vi "Exam.vi"() -> ()   [LabVIEW 2018]
uses:
  <vilib>/DAQmx/write.llb/DAQmx Write (Analog Wfm 1Chan NSamp).vi
  <vilib>/DAQmx/read.llb/DAQmx Read (Analog Wfm 1Chan NSamp).vi
  <vilib>/DAQmx/create/channels.llb/DAQmx Create Channel (AI-Voltage-Basic).vi
  <vilib>/DAQmx/configure/timing.llb/DAQmx Timing (Sample Clock).vi
  <vilib>/DAQmx/miscellaneous.llb/DAQmx Fill In Error Info.vi
  <vilib>/DAQmx/create/channels.llb/DAQmx Create Channel (AO-Voltage-Basic).vi
  <vilib>/measure/NI_MABase.lvlib
panel:
  in  "정지 2":bool
  out "웨이브폼 차트 2":waveform(dbl)(graph)
  out "웨이브폼 차트":waveform(dbl)(graph)
  in  "정지":bool
  in  "정지":bool
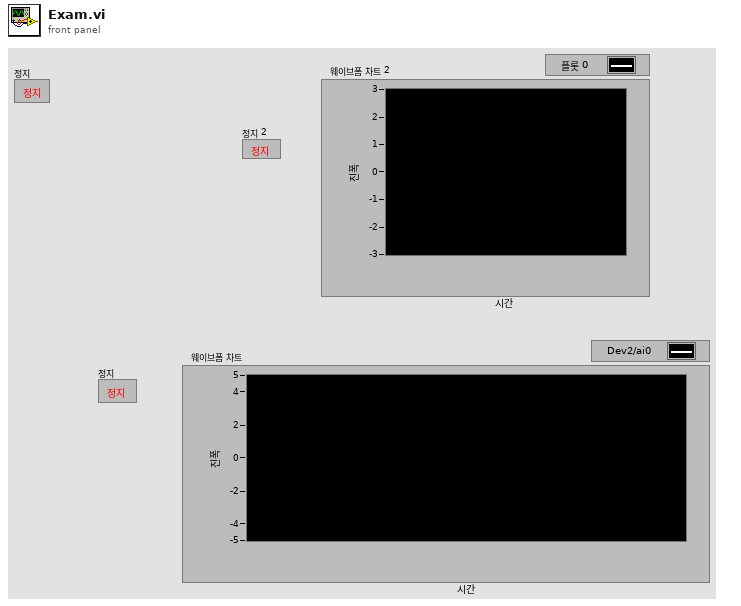
[diagram p1: front panel]
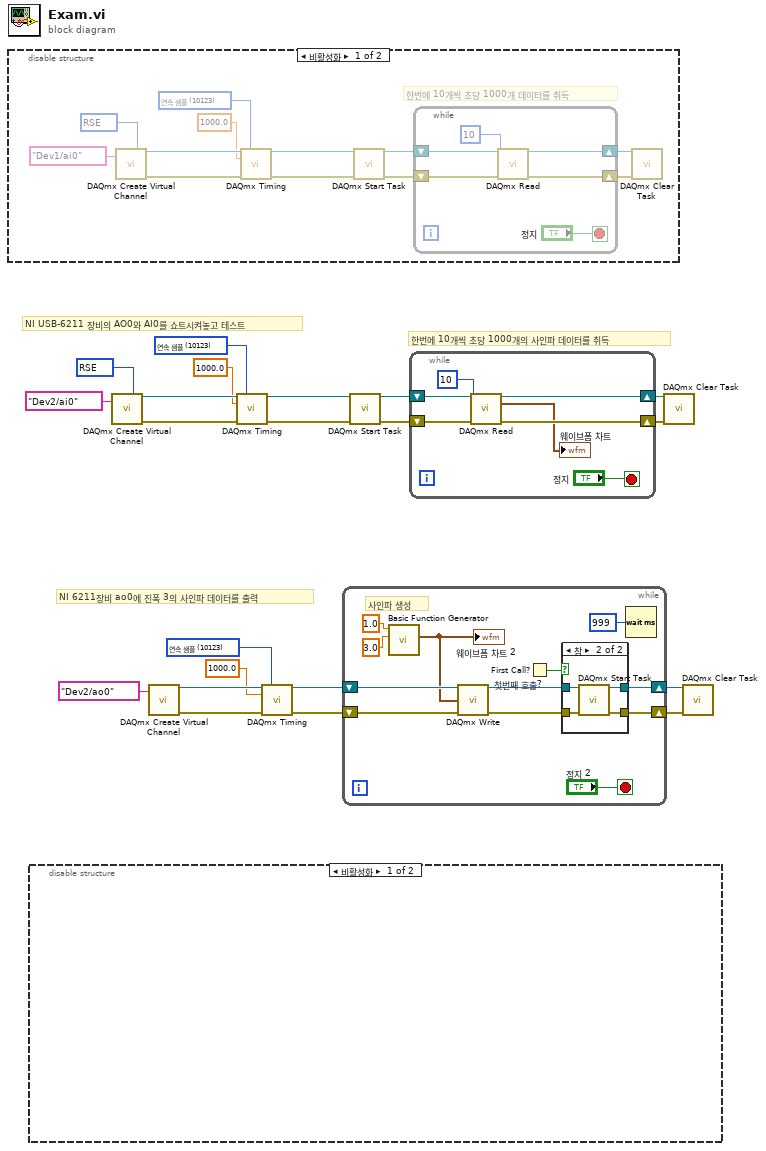
[diagram p0: block diagram]
diagram:
  w1 = 10123 items=["유한 샘플"=10178, "연속 샘플"=10123, "하드웨어 타이밍에 의한 단일 포인트"=12522] ("sample mode")
  w10 = 10123 items=["유한 샘플"=10178, "연속 샘플"=10123, "하드웨어 타이밍에 의한 단일 포인트"=12522] ("sample mode")
  w12 = 10083 items=["기본"=-1, "RSE"=10083, "NRSE"=10078, "차동"=10106, "유사 차동"=12529] ("input terminal configuration")
  # "NI 6211장비 ao0에 진폭 3의 사인파 데이터를 출력"
  # "NI USB-6211 장비의 AO0와 AI0를 쇼트시켜놓고 테스트"
  # "한번에 10개씩 초당 1000개의 사인파 데이터를 취득"
  n1 = disable-structure shown="비활성화" {
    frame Disabled {
      w22 = 10123 items=["유한 샘플"=10178, "연속 샘플"=10123, "하드웨어 타이밍에 의한 단일 포인트"=12522] ("sample mode")
      w24 = 10083 items=["기본"=-1, "RSE"=10083, "NRSE"=10078, "차동"=10106, "유사 차동"=12529] ("input terminal configuration")
      # "한번에 10개씩 초당 1000개 데이터를 취득"
      n2 = call-poly <vilib>:"DAQmx Create Virtual Channel.vi"("input terminal configuration"=w24, "physical channels"=tag "Dev1/ai0") -> ("task out"=w33:refnum<k21>, "error out"=w32:errorcluster)  [unwired: 12 in]
      n3 = call-poly <vilib>:"DAQmx Timing.vi"("task/channels in"=w33, "sample mode"=w22, "rate"=1000.0, "error in"=w32) -> ("task out"=w31:refnum<k21>, "error out"=w30:errorcluster)  [unwired: 10 in]
      n4 = call <vilib>:"DAQmx Start Task.vi"("task/channels in"=w31, "error in"=w30) -> ("task out"=w29:refnum<k21>, "error out"=w28:errorcluster)  [unwired: 12 in]
      n5 = while {
        shift-right: [w37] -> w27
        shift-left: w29 -> [w39]
        shift-right: [w36] -> w26
        shift-left: w28 -> [w38]
        stop <- "정지" stop-if-true
        n6 = call-poly <vilib>:"DAQmx Read.vi"("task/channels in"=w39, "number of samples per channel"=10, "error in"=w38) -> ("task out"=w37:refnum<k21>, "error out"=w36:errorcluster)  [unwired: 10 in, 1 out]
      }
      n7 = call <vilib>:"DAQmx Clear Task.vi"("task in"=w27, "error in"=w26) -> ()  [unwired: 13 in, 1 out]
    }
    frame Enabled {
    }
  }
  n8 = disable-structure shown="비활성화" {
    frame Disabled {
    }
    frame Enabled {
    }
  }
  n9 = call-poly <vilib>:"DAQmx Create Virtual Channel.vi"("input terminal configuration"=w12, "physical channels"=tag "Dev2/ai0") -> ("task out"=w21:refnum<k21>, "error out"=w20:errorcluster)  [unwired: 12 in]
  n10 = call-poly <vilib>:"DAQmx Create Virtual Channel.vi"("physical channels"=tag "Dev2/ao0") -> ("task out"=w8:refnum<k21>, "error out"=w7:errorcluster)  [unwired: 13 in]
  n11 = call-poly <vilib>:"DAQmx Timing.vi"("task/channels in"=w21, "sample mode"=w10, "rate"=1000.0, "error in"=w20) -> ("task out"=w19:refnum<k21>, "error out"=w18:errorcluster)  [unwired: 10 in]
  n12 = call-poly <vilib>:"DAQmx Timing.vi"("task/channels in"=w8, "sample mode"=w1, "rate"=1000.0, "error in"=w7) -> ("task out"=w6:refnum<k21>, "error out"=w5:errorcluster)  [unwired: 10 in]
  n13 = while {
    shift-right: [w47] -> w4
    shift-left: w6 -> [w51]
    shift-right: [w46] -> w3
    shift-left: w5 -> [w50]
    stop <- "정지 2" stop-if-true
    # "사인파 생성"
    n14 = call <vilib>:"Basic Function Generator.vi"("amplitude"=3.0, "frequency"=1.0) -> ("signal out"=w41:waveform(dbl))  [unwired: 7 in, 2 out]
    "웨이브폼 차트 2" <- w41
    n15 = call-poly <vilib>:"DAQmx Write.vi"("task/channels in"=w51, "data"=w41, "error in"=w50) -> ("task out"=w49:refnum<k21>, "error out"=w48:errorcluster)  [unwired: 10 in, 1 out]
    n16 = First Call? "첫번째 호출?"() -> (First Call?: T/F=w43:bool)
    n17 = case shown="참" w43 {
      tunnel: w49 -> [w53 w57]
      tunnel: w48 -> [w52 w56]
      tunnel: [w53 w55] -> w47
      tunnel: [w52 w54] -> w46
      frame False {
      }
      frame True {
        n18 = call <vilib>:"DAQmx Start Task.vi"("task/channels in"=w57, "error in"=w56) -> ("task out"=w55:refnum<k21>, "error out"=w54:errorcluster)  [unwired: 12 in]
      }
    }
    n19 = Wait (ms)(milliseconds to wait=u32 999 ("대기 시간 (ms)")) -> ()  [unwired: 1 out]
  }
  n20 = call <vilib>:"DAQmx Start Task.vi"("task/channels in"=w19, "error in"=w18) -> ("task out"=w17:refnum<k21>, "error out"=w16:errorcluster)  [unwired: 12 in]
  n21 = while {
    shift-right: [w62] -> w15
    shift-left: w17 -> [w64]
    shift-right: [w61] -> w14
    shift-left: w16 -> [w63]
    stop <- "정지" stop-if-true
    n22 = call-poly <vilib>:"DAQmx Read.vi"("task/channels in"=w64, "number of samples per channel"=10, "error in"=w63) -> ("task out"=w62:refnum<k21>, "data"=→"웨이브폼 차트":waveform(dbl), "error out"=w61:errorcluster)  [unwired: 10 in]
  }
  n23 = call <vilib>:"DAQmx Clear Task.vi"("task in"=w15, "error in"=w14) -> ()  [unwired: 13 in, 1 out]
  n24 = call <vilib>:"DAQmx Clear Task.vi"("task in"=w4, "error in"=w3) -> ()  [unwired: 13 in, 1 out]
